vi "Launch Configurator.vi"() -> ()   [LabVIEW 2023]
uses:
  Configuration UI Actor/Configuration UI Actor.lvclass
  <vilib>/ActorFramework/Stop Msg/Stop Msg.lvclass
  IConfiguration UI Actor/IConfiguration UI Actor Messages/Set Virt Instr CFG Msg/Set Virt Instr CFG Msg.lvclass
  IConfiguration UI Actor/IConfiguration UI Actor Messages/Add Instr CFG Msg/Add Instr CFG Msg.lvclass
  IConfiguration UI Actor/IConfiguration UI Actor Messages/Set Series CFG Msg/Set Series CFG Msg.lvclass
  <vilib>/MGI/Panel Manager/Panel Actor/Panel Actor/Panel Actor.lvclass
  <vilib>/MGI/Panel Manager/Panel Actor/Panel Actor/Launch Root Panel Window.vi
  HAL/Devices/DAQmx/DIO/DO DAQmx Fixed Freq PWM CFG/DO DAQmx Fixed Freq PWM CFG.lvclass
  HAL/Devices/DAQmx/DIO/DIO DAQmx Simulated CFGs/DO DAQmx PWM Fixed Freq CFG/DO DAQmx Fixed Freq PWM CFG.lvclass
  HAL/Devices/DAQmx/Thermo/Thermometer DAQmx RTD Cont CFG/Thermometer DAQmx RTD Cont CFG.lvclass
  HAL/Devices/Red-y/Configurations/Pressure Control CFG/Red-y Pressure Control CFG.lvclass
  HAL/Devices/DAQmx/AO/AO DAQmx DC CFG/AO DAQmx DC CFG.lvclass
  HAL/Devices/Red-y/Configurations/Pressure Control CFG Simulated/Red-y Pressure Control CFG Simulated.lvclass
  gitlab/imponator-series-actor/Imponator Wiring Test Actor/Imponator Wiring Test Actor/Imponator Wiring Test Actor.lvclass
  gitlab/imponator-series-actor/Imponator Series Actor/Imponator Series UI Actor/Imponator Series UI Actor.lvclass
  HAL/Devices/DAQmx/AI/AI Current DAQmx Cont CFG/AI Current DAQmx Cont CFG.lvclass
  HAL/Devices/DAQmx/AI/AI Voltage DAQmx Cont CFG/AI Voltage DAQmx Cont CFG.lvclass
  HAL/Devices/DAQmx/AO/AO DAQmx DC Simulated CFG/AO DAQmx DC Simulated CFG.lvclass
  HAL/Devices/DAQmx/AI/AI Current DAQmx Cont CFG Simulated/AI Current DAQmx Cont CFG Simulated.lvclass
panel:
  in  "Add Series":bool
  in  "Add Virt Instr":bool
  in  "Stop":bool
  in  "Add Instr":bool
  out "error out":errorcluster
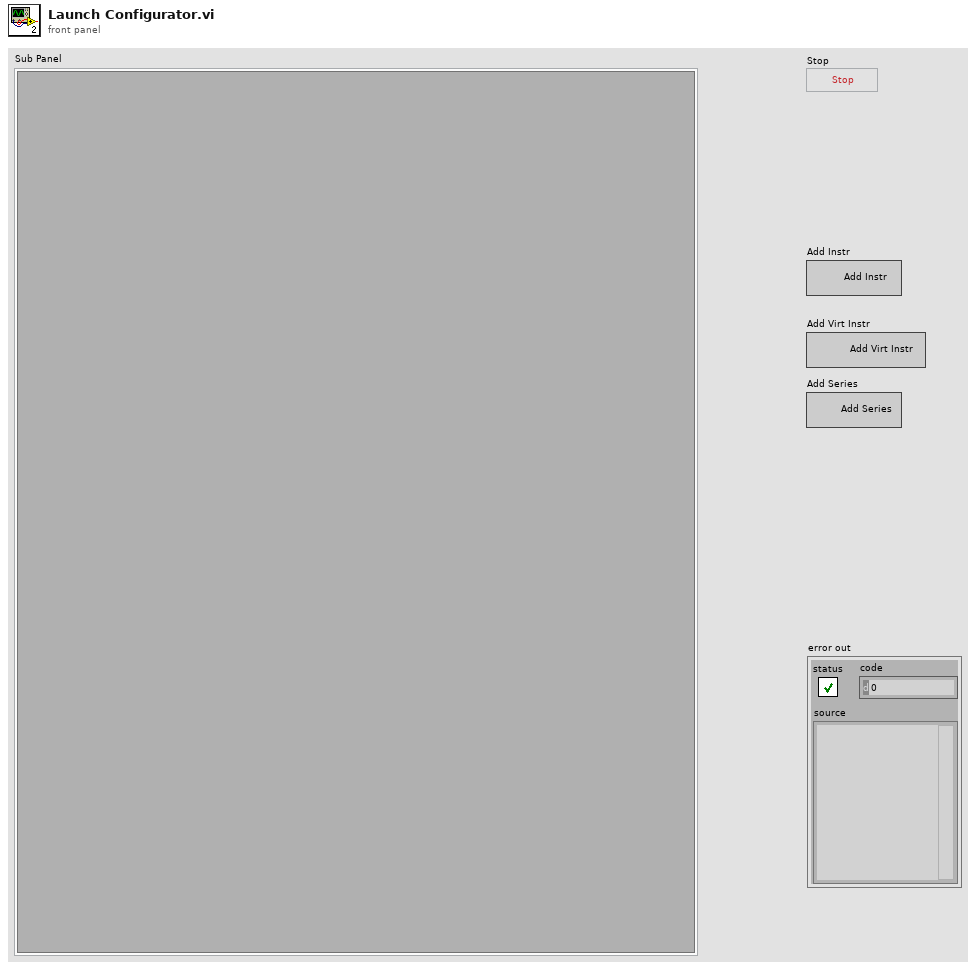
[diagram p1: front panel]
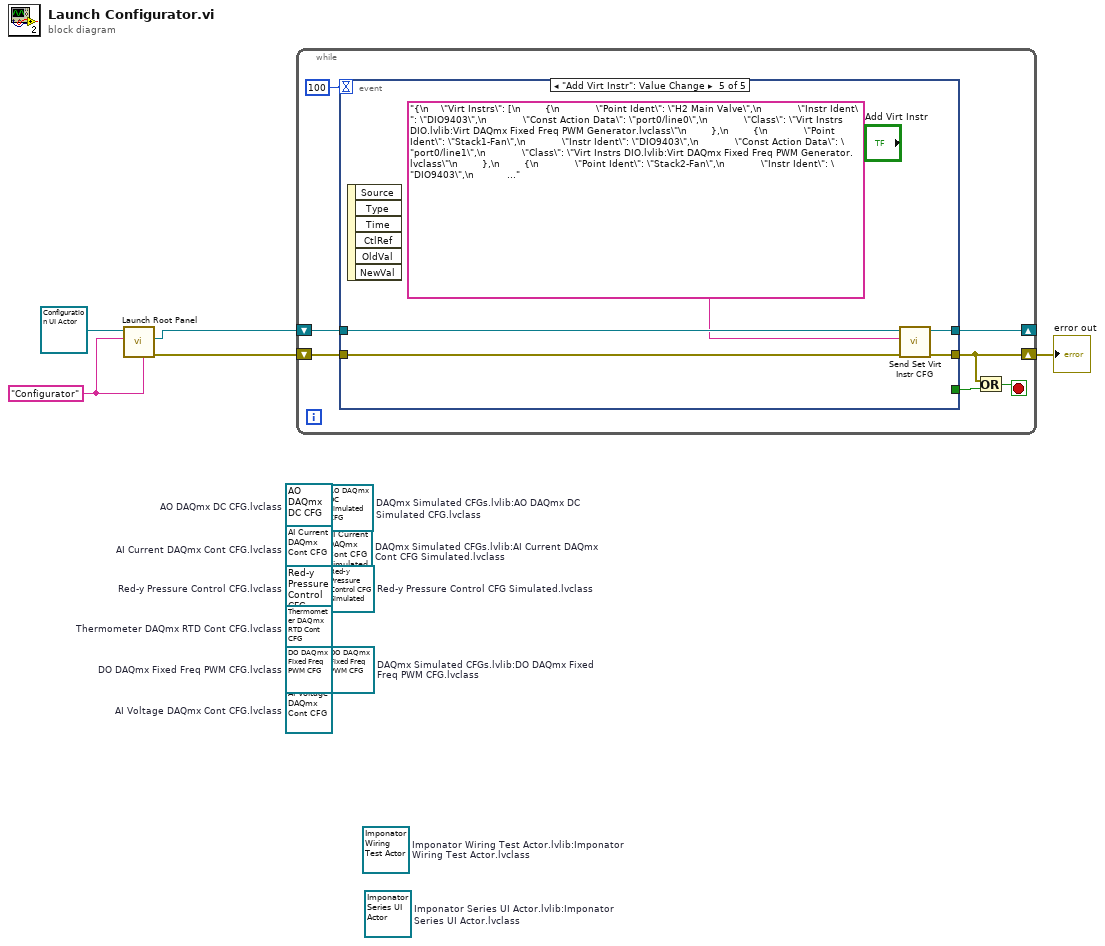
[diagram p0: block diagram]
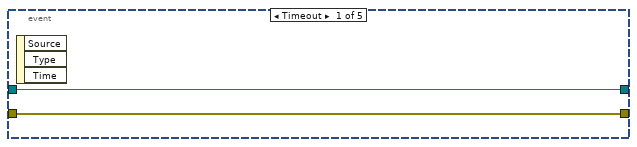
[diagram p2: hidden frame]
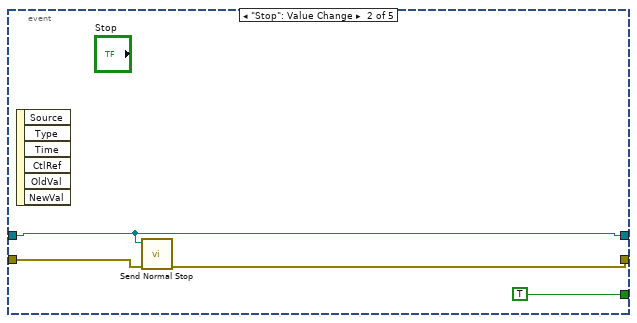
[diagram p3: hidden frame]
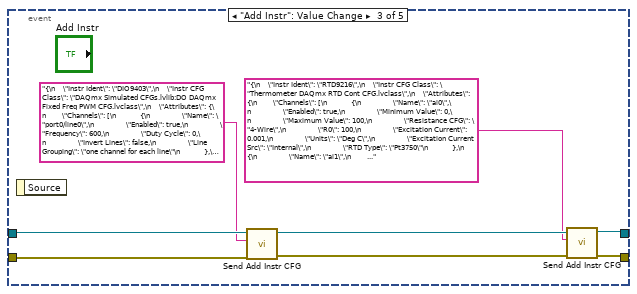
[diagram p4: hidden frame]
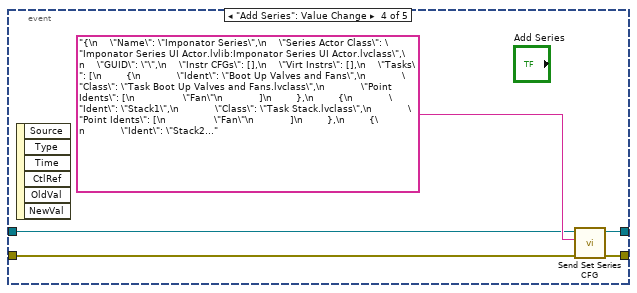
[diagram p5: hidden frame]
diagram:
  (unwired) refnum<class "AI Current DAQmx Cont CFG Simulated.lvclass"> refnum  # DAQmx Simulated CFGs.lvlib:AI Current DAQmx Cont CFG Simulated.lvclass
  (unwired) refnum<class "AO DAQmx DC Simulated CFG.lvclass"> refnum  # DAQmx Simulated CFGs.lvlib:AO DAQmx DC Simulated CFG.lvclass
  (unwired) refnum<class "AI Voltage DAQmx Cont CFG.lvclass"> refnum  # AI Voltage DAQmx Cont CFG.lvclass
  (unwired) refnum<class "Imponator Series UI Actor.lvclass"> refnum  # Imponator Series UI Actor.lvlib:Imponator Series UI Actor.lvclass
  (unwired) refnum<class "Imponator Wiring Test Actor.lvclass"> refnum  # Imponator Wiring Test Actor.lvlib:Imponator Wiring Test Actor.lvclass
  (unwired) refnum<class "Red-y Pressure Control CFG Simulated.lvclass"> refnum  # Red-y Pressure Control CFG Simulated.lvclass
  (unwired) refnum<class "AO DAQmx DC CFG.lvclass"> refnum  # AO DAQmx DC CFG.lvclass
  (unwired) refnum<class "AI Current DAQmx Cont CFG.lvclass"> refnum  # AI Current DAQmx Cont CFG.lvclass
  (unwired) refnum<class "Red-y Pressure Control CFG.lvclass"> refnum  # Red-y Pressure Control CFG.lvclass
  (unwired) refnum<class "Thermometer DAQmx RTD Cont CFG.lvclass"> refnum  # Thermometer DAQmx RTD Cont CFG.lvclass
  (unwired) refnum<class "DO DAQmx Fixed Freq PWM CFG.lvclass"> refnum  # DAQmx Simulated CFGs.lvlib:DO DAQmx Fixed Freq PWM CFG.lvclass
  (unwired) refnum<class "DO DAQmx Fixed Freq PWM CFG.lvclass"> refnum  # DO DAQmx Fixed Freq PWM CFG.lvclass
  w1 = "Configurator" ("Debug Alias")
  n1 = call-poly <vilib>:"Launch Root Panel.vi"("Debug Alias"=w1, "Title"=w1, "Panel Actor in"=refnum<class "Configuration UI Actor.lvclass"> refnum ("Configurator Actor.lvlib:Configurator Actor.lvclass")) -> ("Error Out"=w3:errorcluster, "Actor's Enqueuer"=w4:refnum<class "Message Enqueuer.lvclass">)  [unwired: 7 in]
  n2 = while {
    shift-right: [w8] -> w2
    shift-left: w3 -> [w12]
    shift-right: [w10] -> _
    shift-left: w4 -> [w11]
    stop <- w9 stop-if-true
    n3 = event shown="[4] \"Add Virt Instr\": Value Change" {
      selector: _ -> [_ _ _ _ _]
      dyn-events: _ -> [_ _ _ _ _]
      timeout: 100 -> [_ _ _ _ _]
      tunnel: w12 -> [w14 w18 w25 w28 w36]
      tunnel: [w14 w17 w21 w31 w34] -> w8
      tunnel: w11 -> [w13 w15 w26 w29 w35]
      tunnel: [w13 w15 w20 w27 w33] -> w10
      tunnel: [_ TRUE _ _ _] -> w6
      event Timeout {
        n4 = event-data() -> ()  [unwired: 1 in, 3 out]
      }
      event "Stop": Value Change {
        n5 = event-data() -> ()  [unwired: 1 in, 6 out]
        n6 = call <vilib>:"Send Normal Stop.vi"("error in (no error)"=w18, "Message Enqueuer"=w15) -> ("error out"=w17:errorcluster)  [unwired: 9 in]
      }
      event "Add Instr": Value Change {
        n7 = event-data() -> ()  [unwired: 1 in, 1 out]
        n8 = call "Send Add Instr CFG.vi"("error in (no error)"=w25, "Instr Configuration"="{\n    \"Instr Ident\": \"DIO9403\",\n    \"Instr CFG Class\": \"DAQmx Simulated CFGs.lvlib:DO DAQmx Fixed Freq PWM CFG.lvclass\",\n    \"Attributes\": {\n        \"Channels\": [\n            {\n                \"Name\": \"port0/line0\",\n                \"Enabled\": true,\n                \"Frequency\": 600,\n                \"Duty Cycle\": 0,\n                \"Invert Lines\": false,\n                \"Line Grouping\": \"one channel for each line\"\n            },\n            {\n                \"Name\": \"port0/line1\",\n                \"Enabled\": false,\n                \"Frequency\": 1000,\n                \"Duty Cycle\": 0,\n                \"Invert Lines\": false,\n                \"Line Grouping\": \"one channel for each line\"\n            },\n            {\n                \"Name\": \"port0/line2\",\n                \"Enabled\": true,\n                \"Frequency\": 1000,\n                \"Duty Cycle\": 0,\n                \"Invert Lines\": false,\n                \"Line Grouping\": \"one channel for each line\"\n            },\n            {\n                \"Name\": \"port0/line3\",\n                \"Enabled\": true,\n                \"Frequency\": 1000,\n                \"Duty Cycle\": 0,\n                \"Invert Lines\": false,\n                \"Line Grouping\": \"one channel for each line\"\n            },\n            {\n                \"Name\": \"port0/line4\",\n                \"Enabled\": true,\n                \"Frequency\": 1000,\n                \"Duty Cycle\": 0,\n                \"Invert Lines\": false,\n                \"Line Grouping\": \"one channel for each line\"\n            },\n            {\n                \"Name\": \"port0/line5\",\n                \"Enabled\": true,\n                \"Frequency\": 1000,\n                \"Duty Cycle\": 0,\n                \"Invert Lines\": false,\n                \"Line Grouping\": \"one channel for each line\"\n            },\n            {\n                \"Name\": \"port0/line6\",\n                \"Enabled\": true,\n                \"Frequency\": 1000,\n                \"Duty Cycle\": 0,\n                \"Invert Lines\": false,\n                \"Line Grouping\": \"one channel for each line\"\n            },\n            {\n                \"Name\": \"port0/line7\",\n                \"Enabled\": true,\n                \"Frequency\": 600,\n                \"Duty Cycle\": 0,\n                \"Invert Lines\": false,\n                \"Line Grouping\": \"one channel for each line\"\n            },\n            {\n                \"Name\": \"port0/line8\",\n                \"Enabled\": true,\n                \"Frequency\": 600,\n                \"Duty Cycle\": 0,\n                \"Invert Lines\": false,\n                \"Line Grouping\": \"one channel for each line\"\n            },\n            {\n                \"Name\": \"port0/line9\",\n                \"Enabled\": true,\n                \"Frequency\": 600,\n                \"Duty Cycle\": 0,\n                \"Invert Lines\": false,\n                \"Line Grouping\": \"one channel for each line\"\n            },\n            {\n                \"Name\": \"port0/line10\",\n                \"Enabled\": true,\n                \"Frequency\": 600,\n                \"Duty Cycle\": 0,\n                \"Invert Lines\": false,\n                \"Line Grouping\": \"one channel for each line\"\n            },\n            {\n                \"Name\": \"port0/line11\",\n                \"Enabled\": true,\n                \"Frequency\": 600,\n                \"Duty Cycle\": 0,\n                \"Invert Lines\": false,\n                \"Line Grouping\": \"one channel for each line\"\n            },\n            {\n                \"Name\": \"port0/line12\",\n                \"Enabled\": true,\n                \"Frequency\": 600,\n                \"Duty Cycle\": 0,\n                \"Invert Lines\": false,\n                \"Line Grouping\": \"one channel for each line\"\n            },\n            {\n                \"Name\": \"port0/line13\",\n                \"Enabled\": true,\n                \"Frequency\": 600,\n                \"Duty Cycle\": 0,\n                \"Invert Lines\": false,\n                \"Line Grouping\": \"one channel for each line\"\n            },\n            {\n                \"Name\": \"port0/line14\",\n                \"Enabled\": true,\n                \"Frequency\": 600,\n                \"Duty Cycle\": 0,\n                \"Invert Lines\": false,\n                \"Line Grouping\": \"one channel for each line\"\n            },\n            {\n                \"Name\": \"port0/line15\",\n                \"Enabled\": true,\n                \"Frequency\": 600,\n                \"Duty Cycle\": 0,\n                \"Invert Lines\": false,\n                \"Line Grouping\": \"one channel for each line\"\n            },\n            {\n                \"Name\": \"port0/line16\",\n                \"Enabled\": true,\n                \"Frequency\": 600,\n                \"Duty Cycle\": 0,\n                \"Invert Lines\": false,\n                \"Line Grouping\": \"one channel for each line\"\n            },\n            {\n                \"Name\": \"port0/line17\",\n                \"Enabled\": true,\n                \"Frequency\": 600,\n                \"Duty Cycle\": 0,\n                \"Invert Lines\": false,\n                \"Line Grouping\": \"one channel for each line\"\n            },\n            {\n                \"Name\": \"port0/line18\",\n                \"Enabled\": true,\n                \"Frequency\": 600,\n                \"Duty Cycle\": 0,\n                \"Invert Lines\": false,\n                \"Line Grouping\": \"one channel for each line\"\n            }\n        ],\n        \"Timing\": {\n            \"Mode\": \"Sample Clock\",\n            \"Samples per Channel\": 10000,\n            \"Sample Mode\": \"Continuous Samples\",\n            \"Sample Rate\": 100000,\n            \"Sample Clock Source\": \"OnboardClock\",\n            \"Active Edge\": \"Rising\"\n        },\n        \"Trigger\": {\n            \"Trigger Type\": \"No Trigger\"\n        },\n        \"Generation\": {\n            \"Regen Mode\": \"Allow Regeneration\"\n        }\n    }\n}", "Message Enqueuer"=w26) -> ("error out"=w22:errorcluster, "Message Enqueuer out"=w23:refnum<class "Message Enqueuer.lvclass">)  [unwired: 7 in]
        n9 = call "Send Add Instr CFG.vi"("error in (no error)"=w22, "Instr Configuration"="{\n    \"Instr Ident\": \"RTD9216\",\n    \"Instr CFG Class\": \"Thermometer DAQmx RTD Cont CFG.lvclass\",\n    \"Attributes\": {\n        \"Channels\": [\n            {\n                \"Name\": \"ai0\",\n                \"Enabled\": true,\n                \"Minimum Value\": 0,\n                \"Maximum Value\": 100,\n                \"Resistance CFG\": \"4-Wire\",\n                \"R0\": 100,\n                \"Excitation Current\": 0.001,\n                \"Units\": \"Deg C\",\n                \"Excitation Current Src\": \"Internal\",\n                \"RTD Type\": \"Pt3750\"\n            },\n            {\n                \"Name\": \"ai1\",\n                \"Enabled\": true,\n                \"Minimum Value\": 0,\n                \"Maximum Value\": 100,\n                \"Resistance CFG\": \"3-Wire\",\n                \"R0\": 100,\n                \"Excitation Current\": 0.001,\n                \"Units\": \"Deg C\",\n                \"Excitation Current Src\": \"Internal\",\n                \"RTD Type\": \"Pt3750\"\n            },\n            {\n                \"Name\": \"ai2\",\n                \"Enabled\": true,\n                \"Minimum Value\": 0,\n                \"Maximum Value\": 100,\n                \"Resistance CFG\": \"4-Wire\",\n                \"R0\": 100,\n                \"Excitation Current\": 0.001,\n                \"Units\": \"Deg C\",\n                \"Excitation Current Src\": \"Internal\",\n                \"RTD Type\": \"Pt3750\"\n            },\n            {\n                \"Name\": \"ai3\",\n                \"Enabled\": true,\n                \"Minimum Value\": 0,\n                \"Maximum Value\": 100,\n                \"Resistance CFG\": \"4-Wire\",\n                \"R0\": 100,\n                \"Excitation Current\": 0.001,\n                \"Units\": \"Deg C\",\n                \"Excitation Current Src\": \"Internal\",\n                \"RTD Type\": \"Pt3750\"\n            },\n            {\n                \"Name\": \"ai4\",\n                \"Enabled\": true,\n                \"Minimum Value\": 0,\n                \"Maximum Value\": 100,\n                \"Resistance CFG\": \"4-Wire\",\n                \"R0\": 100,\n                \"Excitation Current\": 0.001,\n                \"Units\": \"Deg C\",\n                \"Excitation Current Src\": \"Internal\",\n                \"RTD Type\": \"Pt3750\"\n            },\n            {\n                \"Name\": \"ai5\",\n                \"Enabled\": true,\n                \"Minimum Value\": 0,\n                \"Maximum Value\": 100,\n                \"Resistance CFG\": \"4-Wire\",\n                \"R0\": 100,\n                \"Excitation Current\": 0.001,\n                \"Units\": \"Deg C\",\n                \"Excitation Current Src\": \"Internal\",\n                \"RTD Type\": \"Pt3750\"\n            },\n            {\n                \"Name\": \"ai6\",\n                \"Enabled\": false,\n                \"Minimum Value\": 0,\n                \"Maximum Value\": 100,\n                \"Resistance CFG\": \"4-Wire\",\n                \"R0\": 100,\n                \"Excitation Current\": 0.001,\n                \"Units\": \"Deg C\",\n                \"Excitation Current Src\": \"Internal\",\n                \"RTD Type\": \"Pt3750\"\n            },\n            {\n                \"Name\": \"ai7\",\n                \"Enabled\": false,\n                \"Minimum Value\": 0,\n                \"Maximum Value\": 100,\n                \"Resistance CFG\": \"4-Wire\",\n                \"R0\": 100,\n                \"Excitation Current\": 0.001,\n                \"Units\": \"Deg C\",\n                \"Excitation Current Src\": \"Internal\",\n                \"RTD Type\": \"Pt3750\"\n            }\n        ],\n        \"Timing\": {\n            \"Mode\": \"Sample Clock\",\n            \"Samples per Channel\": 1000,\n            \"Sample Mode\": \"Continuous Samples\",\n            \"Sample Rate\": 10,\n            \"Sample Clock Source\": \"OnboardClock\",\n            \"Active Edge\": \"Rising\"\n        },\n        \"Trigger\": {\n            \"Trigger Type\": \"No Trigger\"\n        }\n    }\n}", "Message Enqueuer"=w23) -> ("error out"=w21:errorcluster, "Message Enqueuer out"=w20:refnum<class "Message Enqueuer.lvclass">)  [unwired: 7 in]
      }
      event "Add Series": Value Change {
        n10 = event-data() -> ()  [unwired: 1 in, 6 out]
        n11 = call "Send Set Series CFG.vi"("error in (no error)"=w28, "Series CFG"="{\n    \"Name\": \"Imponator Series\",\n    \"Series Actor Class\": \"Imponator Series UI Actor.lvlib:Imponator Series UI Actor.lvclass\",\n    \"GUID\": \"\",\n    \"Instr CFGs\": [],\n    \"Virt Instrs\": [],\n    \"Tasks\": [\n        {\n            \"Ident\": \"Boot Up Valves and Fans\",\n            \"Class\": \"Task Boot Up Valves and Fans.lvclass\",\n            \"Point Idents\": [\n                \"Fan\"\n            ]\n        },\n        {\n            \"Ident\": \"Stack1\",\n            \"Class\": \"Task Stack.lvclass\",\n            \"Point Idents\": [\n                \"Fan\"\n            ]\n        },\n        {\n            \"Ident\": \"Stack2\",\n            \"Class\": \"Task Stack.lvclass\",\n            \"Point Idents\": [\n                \"Fan\"\n            ]\n        },\n        {\n            \"Ident\": \"Stack3\",\n            \"Class\": \"Task Stack.lvclass\",\n            \"Point Idents\": [\n                \"Fan\"\n            ]\n        },\n        {\n            \"Ident\": \"Stack4\",\n            \"Class\": \"Task Stack.lvclass\",\n            \"Point Idents\": [\n                \"Fan\"\n            ]\n        },\n        {\n            \"Ident\": \"Stack5\",\n            \"Class\": \"Task Stack.lvclass\",\n            \"Point Idents\": [\n                \"Fan\"\n            ]\n        },\n        {\n            \"Ident\": \"Stack6\",\n            \"Class\": \"Task Stack.lvclass\",\n            \"Point Idents\": [\n                \"Fan\"\n            ]\n        }\n    ]\n}", "Message Enqueuer"=w29) -> ("error out"=w31:errorcluster, "Message Enqueuer out"=w27:refnum<class "Message Enqueuer.lvclass">)  [unwired: 7 in]
      }
      event "Add Virt Instr": Value Change {
        n12 = event-data() -> ()  [unwired: 1 in, 6 out]
        n13 = call "Send Set Virt Instr CFG.vi"("error in (no error)"=w36, "Virt Instr CFG"="{\n    \"Virt Instrs\": [\n        {\n            \"Point Ident\": \"H2 Main Valve\",\n            \"Instr Ident\": \"DIO9403\",\n            \"Const Action Data\": \"port0/line0\",\n            \"Class\": \"Virt Instrs DIO.lvlib:Virt DAQmx Fixed Freq PWM Generator.lvclass\"\n        },\n        {\n            \"Point Ident\": \"Stack1-Fan\",\n            \"Instr Ident\": \"DIO9403\",\n            \"Const Action Data\": \"port0/line1\",\n            \"Class\": \"Virt Instrs DIO.lvlib:Virt DAQmx Fixed Freq PWM Generator.lvclass\"\n        },\n        {\n            \"Point Ident\": \"Stack2-Fan\",\n            \"Instr Ident\": \"DIO9403\",\n            \"Const Action Data\": \"port0/line2\",\n            \"Class\": \"Virt Instrs DIO.lvlib:Virt DAQmx Fixed Freq PWM Generator.lvclass\"\n        },\n        {\n            \"Point Ident\": \"Stack3-Fan\",\n            \"Instr Ident\": \"DIO9403\",\n            \"Const Action Data\": \"port0/line3\",\n            \"Class\": \"Virt Instrs DIO.lvlib:Virt DAQmx Fixed Freq PWM Generator.lvclass\"\n        },\n        {\n            \"Point Ident\": \"Stack4-Fan\",\n            \"Instr Ident\": \"DIO9403\",\n            \"Const Action Data\": \"port0/line4\",\n            \"Class\": \"Virt Instrs DIO.lvlib:Virt DAQmx Fixed Freq PWM Generator.lvclass\"\n        },\n        {\n            \"Point Ident\": \"Stack5-Fan\",\n            \"Instr Ident\": \"DIO9403\",\n            \"Const Action Data\": \"port0/line5\",\n            \"Class\": \"Virt Instrs DIO.lvlib:Virt DAQmx Fixed Freq PWM Generator.lvclass\"\n        },\n        {\n            \"Point Ident\": \"Stack6-Fan\",\n            \"Instr Ident\": \"DIO9403\",\n            \"Const Action Data\": \"port0/line6\",\n            \"Class\": \"Virt Instrs DIO.lvlib:Virt DAQmx Fixed Freq PWM Generator.lvclass\"\n        },\n        {\n            \"Point Ident\": \"Stack1-H2 Valve\",\n            \"Instr Ident\": \"DIO9403\",\n            \"Const Action Data\": \"port0/line7\",\n            \"Class\": \"Virt Instrs DIO.lvlib:Virt DAQmx Fixed Freq PWM Generator.lvclass\"\n        },\n        {\n            \"Point Ident\": \"Stack2-H2 Valve\",\n            \"Instr Ident\": \"DIO9403\",\n            \"Const Action Data\": \"port0/line8\",\n            \"Class\": \"Virt Instrs DIO.lvlib:Virt DAQmx Fixed Freq PWM Generator.lvclass\"\n        },\n        {\n            \"Point Ident\": \"Stack3-H2 Valve\",\n            \"Instr Ident\": \"DIO9403\",\n            \"Const Action Data\": \"port0/line9\",\n            \"Class\": \"Virt Instrs DIO.lvlib:Virt DAQmx Fixed Freq PWM Generator.lvclass\"\n        },\n        {\n            \"Point Ident\": \"Stack4-H2 Valve\",\n            \"Instr Ident\": \"DIO9403\",\n            \"Const Action Data\": \"port0/line10\",\n            \"Class\": \"Virt Instrs DIO.lvlib:Virt DAQmx Fixed Freq PWM Generator.lvclass\"\n        },\n        {\n            \"Point Ident\": \"Stack5-H2 Valve\",\n            \"Instr Ident\": \"DIO9403\",\n            \"Const Action Data\": \"port0/line11\",\n            \"Class\": \"Virt Instrs DIO.lvlib:Virt DAQmx Fixed Freq PWM Generator.lvclass\"\n        },\n        {\n            \"Point Ident\": \"Stack6-H2 Valve\",\n            \"Instr Ident\": \"DIO9403\",\n            \"Const Action Data\": \"port0/line12\",\n            \"Class\": \"Virt Instrs DIO.lvlib:Virt DAQmx Fixed Freq PWM Generator.lvclass\"\n        },\n        {\n            \"Point Ident\": \"Stack1-Switch\",\n            \"Instr Ident\": \"DIO9403\",\n            \"Const Action Data\": \"port0/line13\",\n            \"Class\": \"Virt Instrs DIO.lvlib:Virt DAQmx Fixed Freq PWM Generator.lvclass\"\n        },\n        {\n            \"Point Ident\": \"Stack2-Switch\",\n            \"Instr Ident\": \"DIO9403\",\n            \"Const Action Data\": \"port0/line14\",\n            \"Class\": \"Virt Instrs DIO.lvlib:Virt DAQmx Fixed Freq PWM Generator.lvclass\"\n        },\n        {\n            \"Point Ident\": \"Stack3-Switch\",\n            \"Instr Ident\": \"DIO9403\",\n            \"Const Action Data\": \"port0/line15\",\n            \"Class\": \"Virt Instrs DIO.lvlib:Virt DAQmx Fixed Freq PWM Generator.lvclass\"\n        },\n        {\n            \"Point Ident\": \"Stack4-Switch\",\n            \"Instr Ident\": \"DIO9403\",\n            \"Const Action Data\": \"port0/line16\",\n            \"Class\": \"Virt Instrs DIO.lvlib:Virt DAQmx Fixed Freq PWM Generator.lvclass\"\n        },\n        {\n            \"Point Ident\": \"Stack5-Switch\",\n            \"Instr Ident\": \"DIO9403\",\n            \"Const Action Data\": \"port0/line17\",\n            \"Class\": \"Virt Instrs DIO.lvlib:Virt DAQmx Fixed Freq PWM Generator.lvclass\"\n        },\n        {\n            \"Point Ident\": \"Stack6-Switch\",\n            \"Instr Ident\": \"DIO9403\",\n            \"Const Action Data\": \"port0/line18\",\n            \"Class\": \"Virt Instrs DIO.lvlib:Virt DAQmx Fixed Freq PWM Generator.lvclass\"\n        },\n        {\n            \"Point Ident\": \"Stack1-Temp\",\n            \"Instr Ident\": \"RTD9216\",\n            \"Const Action Data\": \"ai0\",\n            \"Class\": \"HAL GOOP4.lvlib:Virt Instr Target.lvclass\"\n        },\n        {\n            \"Point Ident\": \"Stack2-Temp\",\n            \"Instr Ident\": \"RTD9216\",\n            \"Const Action Data\": \"ai1\",\n            \"Class\": \"HAL GOOP4.lvlib:Virt Instr Target.lvclass\"\n        },\n        {\n            \"Point Ident\": \"Stack3-Temp\",\n            \"Instr Ident\": \"RTD9216\",\n            \"Const Action Data\": \"ai2\",\n            \"Class\": \"HAL GOOP4.lvlib:Virt Instr Target.lvclass\"\n        },\n        {\n            \"Point Ident\": \"Stack4-Temp\",\n            \"Instr Ident\": \"RTD9216\",\n            \"Const Action Data\": \"ai3\",\n            \"Class\": \"HAL GOOP4.lvlib:Virt Instr Target.lvclass\"\n        },\n        {\n            \"Point Ident\": \"Stack5-Temp\",\n            \"Instr Ident\": \"RTD9216\",\n            \"Const Action Data\": \"ai4\",\n            \"Class\": \"HAL GOOP4.lvlib:Virt Instr Target.lvclass\"\n        },\n        {\n            \"Point Ident\": \"Stack6-Temp\",\n            \"Instr Ident\": \"RTD9216\",\n            \"Const Action Data\": \"ai5\",\n            \"Class\": \"HAL GOOP4.lvlib:Virt Instr Target.lvclass\"\n        }\n    ]\n}", "Message Enqueuer"=w35) -> ("error out"=w34:errorcluster, "Message Enqueuer out"=w33:refnum<class "Message Enqueuer.lvclass">)  [unwired: 7 in]
      }
    }
    n14 = Or(x=w8, y=w6) -> (x .or. y?=w9:bool)
  }
  "error out" <- w2
